vi "gu_copy.vi"(8 "error in":errorcluster, 10 "Destination Path":T1, 11 "Source Path":T1) -> (0 "error out":errorcluster, 3 "result":i32)   [LabVIEW 2020, in "G-Unicode.lvlib"]
uses:
  Types/Encoded UTF-8 String.ctl
  G-Unicode.lvlib
  lib/g_unicode_32.dll
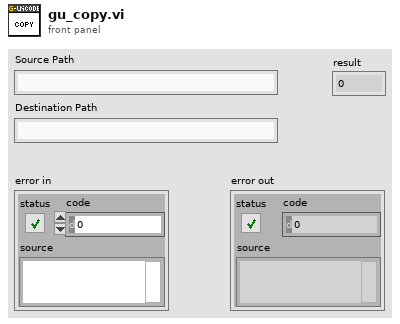
[diagram p1: front panel]
types:
  T1 = typedef "G-Unicode.lvlib/Encoded UTF-8 String.ctl" = string
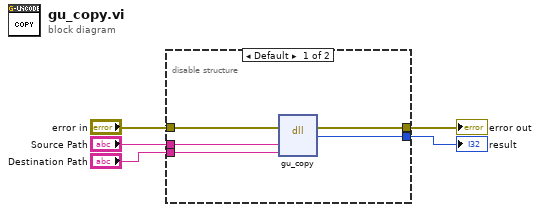
[diagram p0: block diagram]
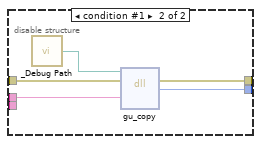
[diagram p2: hidden frame]
diagram:
  n1 = disable-structure shown="Default" {
    disable-tunnel: [w10 w15] -> w5
    disable-tunnel: [w9 w14] -> w4
    disable-tunnel: "Source Path" -> [w8 w13]
    disable-tunnel: "error in" -> [w7 w12]
    disable-tunnel: "Destination Path" -> [w6 _]
    frame condition #0 (active) {
      n2 = dll-call lib="C:/github/dataflowg/g-unicode/src/LabVIEW/G-Unicode/lib/g_unicode_*.*" fn="gu_copy"(error in=w7, "source_path"=w8, "dest_path"=w6) -> (error out=w10:errorcluster, "result"=w9:i32)  [unwired: 4 in, 1 out]
    }
    frame condition #1 {
      n3 = call "_Debug Path.vi"() -> ("Debug Path"=w11:path)
      n4 = dll-call lib="?" fn="gu_copy"(path in=w11, error in=w12, "source_path"=w13) -> (error out=w15:errorcluster, "result"=w14:i32)  [unwired: 4 in, 1 out]
    }
  }
  "error out" <- w5
  "result" <- w4
